vi "Test Helper Loop Broadcast Running State.vi"(8 "error in (no error)":errorcluster, 11 "Helper Loop Test In":refnum<class "Helper Loop Test.lvclass">) -> (0 "error out":errorcluster, 3 "Helper Loop Test Out":refnum<class "Helper Loop Test.lvclass">)   [LabVIEW 2020, in "Helper Loop Test.lvclass"]
uses:
  Helper Loop Test.lvclass
  C:/Program Files (x86)/National Instruments/LabVIEW 2020/vi.lib/Astemes/LUnit/Test Case.lvclass
  source/Framework Test Suite/Mock Process/Mock Process.lvclass
  C:/git/astemes-triarc-framework/source/Framework/Process/Process.lvclass
  <vilib>/Astemes/LUnit/Test Case.lvclass/Test Case.ctl
  source/Framework/Process/Process.lvclass/Process.ctl
  78a70cba-abe8-4254-87f5-2f6725d0919d.vi
  source/Framework/Broadcast Event Dequeuers/Execution timer.vi
  <vilib>/Astemes/LUnit/Append Pass Result.vi
  <vilib>/Astemes/LUnit/Append Fail Result.vi
  78a70cba-abe8-4254-87f5-2f6725d0919d.vi/9c5d11cd-9439-4240-a1ee-d9baace9c924.vi
  source/Framework/Process/Private/SubVIs/Wait for finish.vi
  source/Framework/Process/Private/SubVIs/Set Lifecycle State.vi
  source/Framework/Process/Protected/Messaging/Send Message.vi
  <vilib>/Astemes/LUnit/Run In UI.vi
  source/Framework/Process/Private/SubVIs/Handle Debug Data.vi
  <vilib>/Utility/error.llb/Clear Errors.vi
  source/Framework/Logging/Log Debug.vi
  <vilib>/AdvancedString/1D String Array to Delimited String.vi
  <vilib>/Utility/High Resolution Relative Seconds.vi
  source/Framework/Broadcast Event Dequeuers/Dequeue Broadcast Message.vi
  source/Framework/Process/Public/Lifecycle/Get Lifecycle State.vi
  <vilib>/Utility/error.llb/Error Cluster From Error Code.vi
  source/Framework/Process/Public/Read Name.vi
  source/Framework/Callback/Callback.lvclass
  source/Framework/Process/Process.lvclass
  Helper Loop Test.lvclass/Helper Loop Test.ctl
  source/Framework/Broadcast Event Dequeuers/Broadcast Event Dequeuers.lvlib
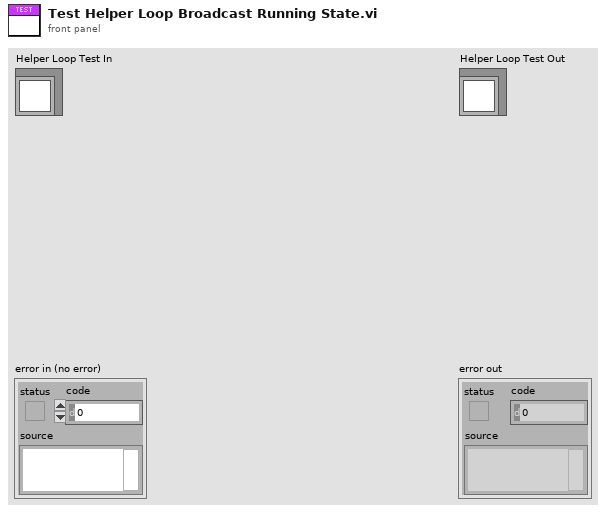
[diagram p1: front panel]
types:
  T1 = cluster{"Message":string, "Message Data":variant}
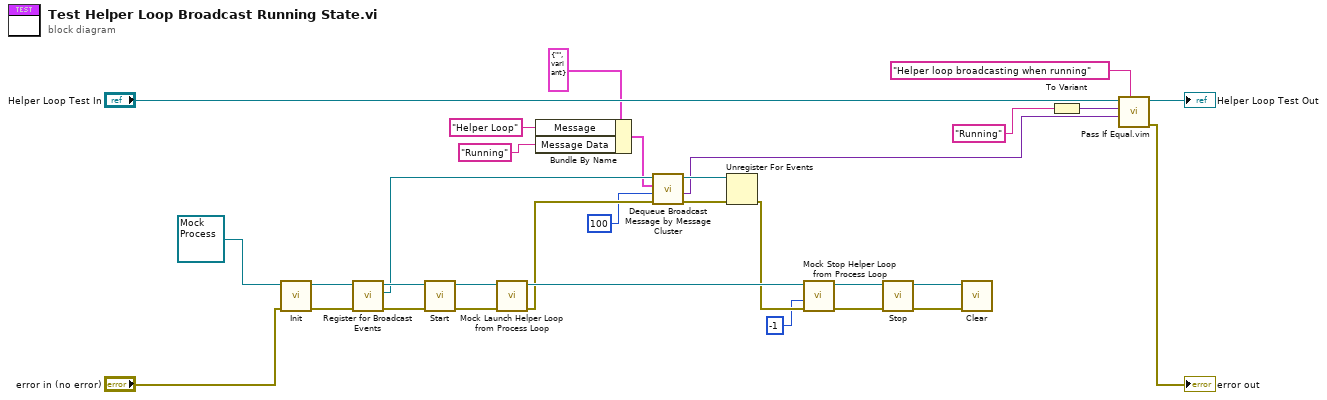
[diagram p0: block diagram]
diagram:
  n1 = call-dynamic "Init.vi"("error in (no error)"="error in (no error)", "Mock Process In"=refnum<class "Mock Process.lvclass"> refnum) -> ("error out"=w29:errorcluster, "Mock Process Out"=w30:refnum<class "Mock Process.lvclass">)  [unwired: 8 in]
  n2 = call "Register for Broadcast Events.vi"("error in (no error)"=w29, "Process In"=w30) -> ("error out"=w27:errorcluster, "Event Registration Refnum Out"=w15:refnum<event-registration>, "Process Out"=w28:refnum<class "Mock Process.lvclass">)  [unwired: 7 in]
  n3 = call "Start.vi"("error in (no error)"=w27, "Process In"=w28) -> ("error out"=w25:errorcluster, "Process Out"=w26:refnum<class "Mock Process.lvclass">)  [unwired: 7 in, 1 out]
  n4 = call "Mock Launch Helper Loop from Process Loop.vi"("error in (no error)"=w25, "Mock Process in"=w26) -> ("error out"=w13:errorcluster, "Mock Process out"=w24:refnum<class "Mock Process.lvclass">)  [unwired: 8 in]
  n5 = Bundle By Name(cluster=T1 {"Message"="", "Message Data"=variant} ("Message"), "Message"="Helper Loop" ("y"), "Message Data"="Running" ("Description")) -> (w4:T1)
  n6 = call "Dequeue Broadcast Message by Message Cluster.vi"("error in (no error)"=w13, "Timeout (-1)"=100, "Message"=w4, "Event Registration Refnum"=w15) -> ("error out"=w9:errorcluster, "Message Data"=w7:variant, "Event Registration Refnum Out"=w8:refnum<event-registration>)  [unwired: 3 in, 2 out]
  n7 = Unregister For Events(event registration refnum=w8, error in=w9) -> (error out=w12:errorcluster)
  n8 = call "Mock Stop Helper Loop from Process Loop.vi"("error in (no error)"=w12, "timeout in ms (-1)"=-1, "Mock Process in"=w24) -> ("error out"=w22:errorcluster, "Mock Process out"=w23:refnum<class "Mock Process.lvclass">)  [unwired: 6 in, 1 out]
  n9 = call "Stop.vi"("error in (no error)"=w22, "Process In"=w23) -> ("error out"=w21:errorcluster, "Process Out"=w10:refnum<class "Mock Process.lvclass">)  [unwired: 7 in, 1 out]
  n10 = call-dynamic "Clear.vi"("error in (no error)"=w21, "Mock Process In"=w10) -> ()  [unwired: 9 in, 1 out]
  n11 = To Variant(anything="Running" ("Description")) -> (Variant=w1:variant)
  n12 = call "Pass If Equal.vim"("Description"="Helper loop broadcasting when running", "Actual"=w7, "Expected"=w1, "LUnit Test Case In"="Helper Loop Test In") -> ("error out"=→"error out":errorcluster, "LUnit Test Case Out"=→"Helper Loop Test Out":refnum<class "Helper Loop Test.lvclass">)  [unwired: 6 in]
